vi "code_facade.vi"(0 "Data In":T4, 2 "Display State In":T2, 3 "Container State":T3) -> (6 "Data Out":T4, 7 "Display State Out":T2, 8 "Action":T1)   [LabVIEW 2022 SP3, in "Code.xctl"]
uses:
  Code.xctl
  code_data.ctl
  <vilib>/_xctls/Container State.ctl
  code_state.ctl
  <vilib>/_xctls/Action.ctl
  <vilib>/event_ctls.llb/eventvkey.ctl
  <vilib>/_xctls/XControlSupport.lvlib
panel:
  out "VKey":T5
  in  "Python Code":string
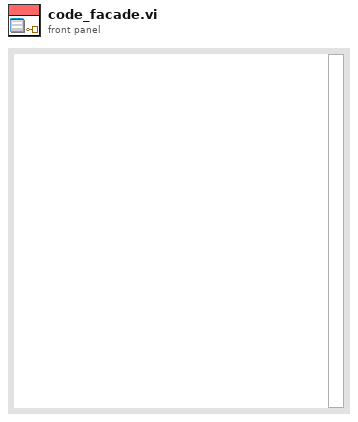
[diagram p1: front panel]
types:
  T1 = typedef "XControlSupport.lvlib/Action.ctl" = cluster{"Data Changed?":bool, "State Changed?":bool, "Action Name":string}
  T2 = typedef "Code.xctl/code_state.ctl" = cluster{"Numeric":dbl}
  T3 = typedef "XControlSupport.lvlib/Container State.ctl" = cluster{"Indicator?":bool, "Run Mode?":bool, " Refnum":refnum<vi>}
  T4 = typedef "Code.xctl/code_data.ctl" = string
  T5 = typedef "eventvkey.ctl" = enum16{"ASCII", "Enter", "Return", "Shift", "Ctrl", "Alt", "Cmd", "Opt", "Caps", "NumLock", "Clear", "Break", "Up", "Down", "Left", "Right", "Insert", "Delete", "Home", "End", "PageUp", "PageDown", "Escape", "Help", "Pause", "ScrollLock", "F1", "F2", "F3", "F4", "F5", "F6", "F7", "F8", "F9", "F10", "F11", "F12", "F13", "F14", "F15", "F16", "F17", "F18", "F19", "F20", "F21", "F22", "F23", "F24", "Play", "VolumeUp", "VolumeDown", "Mute", "Two Byte Char"}
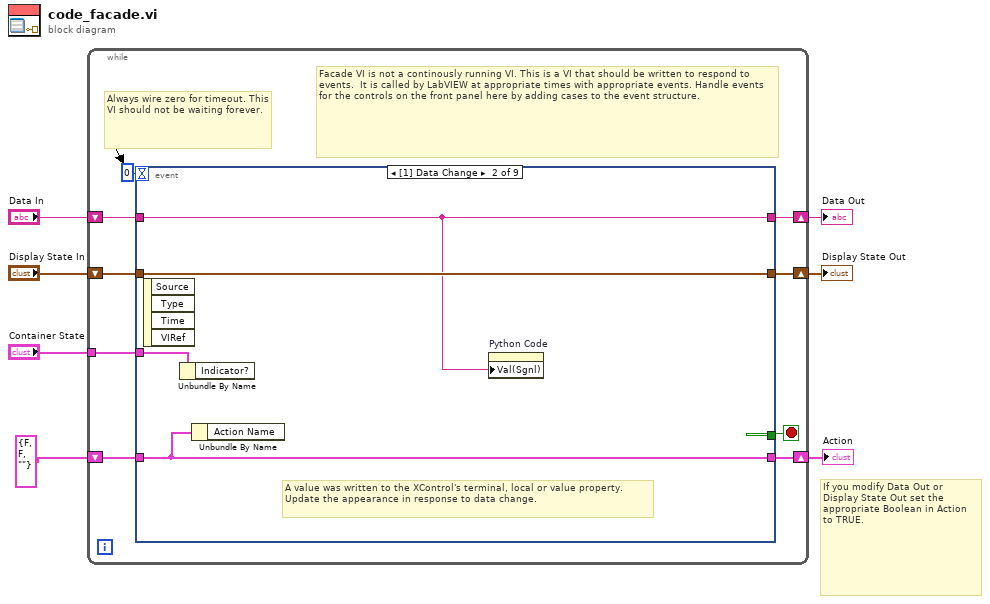
[diagram p0: block diagram]
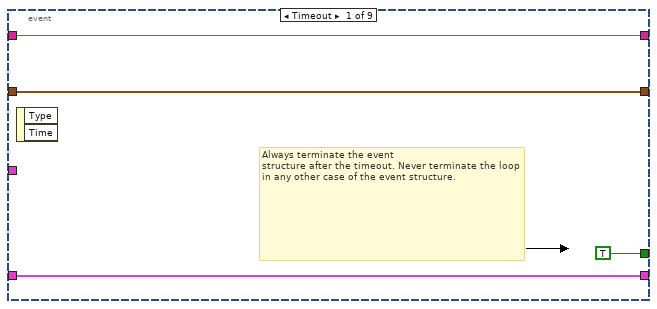
[diagram p2: hidden frame]
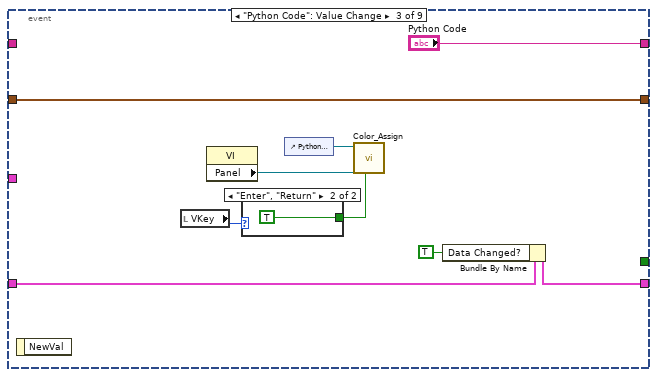
[diagram p3: hidden frame]
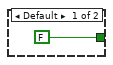
[diagram p4: hidden frame]
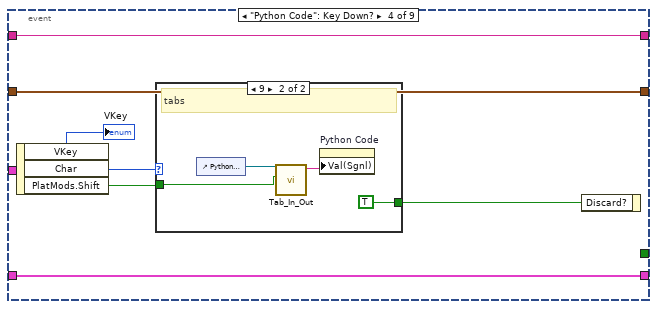
[diagram p5: hidden frame]
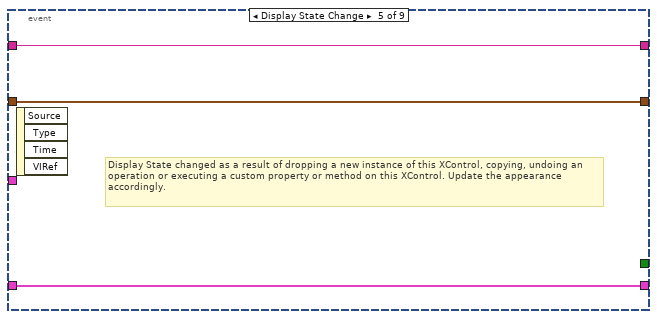
[diagram p7: hidden frame]
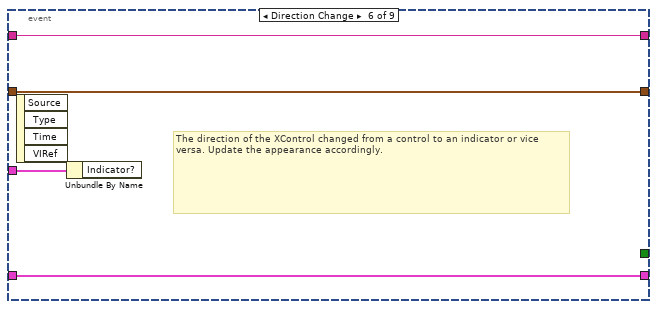
[diagram p8: hidden frame]
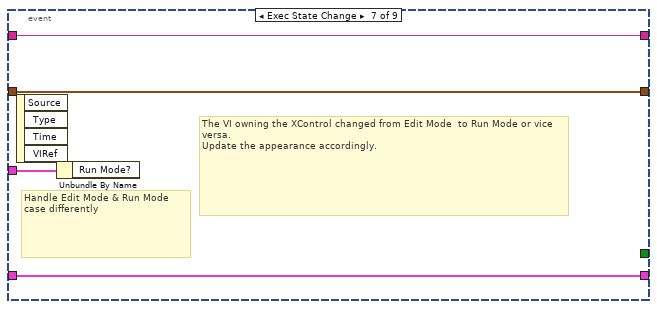
[diagram p9: hidden frame]
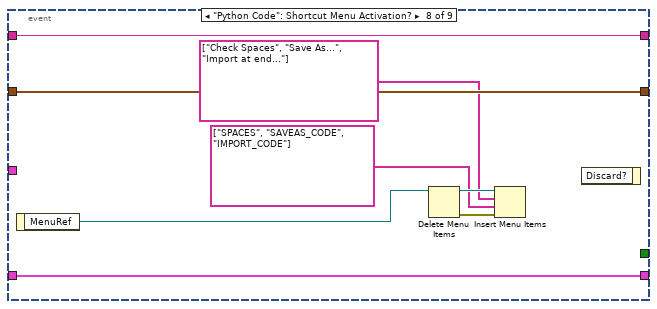
[diagram p10: hidden frame]
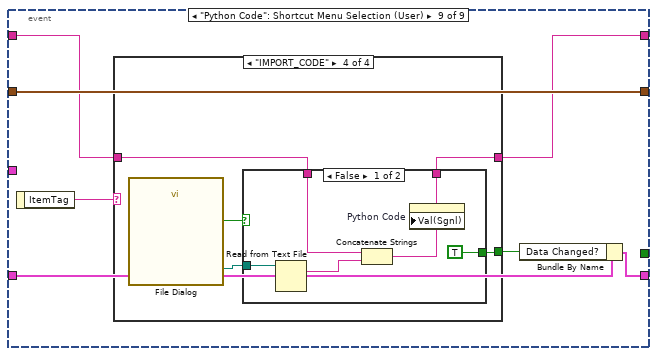
[diagram p11: hidden frame]
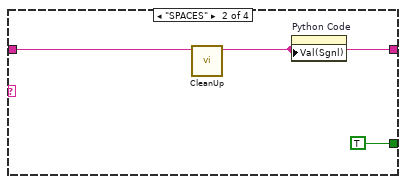
[diagram p13: hidden frame]
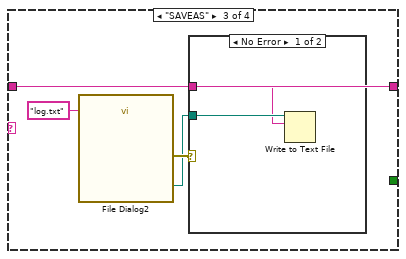
[diagram p14: hidden frame]
diagram:
  # "If you modify Data Out or\nDisplay State Out set the\nappropriate Boolean in Action\nto TRUE."
  n1 = while {
    shift-right: [w15] -> w4
    shift-left: "Display State In" -> [w16]
    tunnel: "Container State" -> [w12]
    shift-right: [w10] -> w7
    shift-left: "Data In" -> [w11]
    shift-right: [w8] -> w2
    shift-left: T1 {"Data Changed?"=FALSE, "State Changed?"=FALSE, "Action Name"=""} ("Action") -> [w9]
    stop <- w14 stop-if-true
    # "Facade VI is not a continously running VI. This is a VI that should be written to respond to events.  It is called by LabVIEW at appropriate times with appropriate events. Handle events for the controls on the front panel here by adding cases to the event structure."
    # "Always wire zero for timeout. This\nVI should not be waiting forever."
    n2 = event shown="[1] Data Change" {
      selector: _ -> [_ _ _ _ _ _ _ _ _]
      dyn-events: _ -> [_ _ _ _ _ _ _ _ _]
      timeout: 0 -> [_ _ _ _ _ _ _ _ _]
      tunnel: w16 -> [w18 w24 w33 w42 w49 w52 w56 w65 w72]
      tunnel: [w18 w24 w33 w42 w49 w52 w56 w65 w72] -> w15
      tunnel: [TRUE _ _ _ _ _ _ _ _] -> w14
      tunnel: w12 -> [_ w23 _ _ _ w53 w57 _ _]
      tunnel: w11 -> [w17 w21 _ w40 w48 w51 w55 w64 w69]
      tunnel: [w17 w21 "Python Code" w40 w48 w51 w55 w64 w70] -> w10
      tunnel: [w19 w22 w30 w41 w47 w50 w54 w63 w67] -> w8
      tunnel: w9 -> [w19 w22 w29 w41 w47 w50 w54 w63 w66]
      event Timeout {
        # "Always terminate the event\nstructure after the timeout. Never terminate the loop in any other case of the event structure."
        n3 = event-data() -> ()  [unwired: 1 in, 2 out]
      }
      event Data Change {
        # "A value was written to the XControl's terminal, local or value property.\nUpdate the appearance in response to data change."
        n4 = event-data() -> ()  [unwired: 1 in, 4 out]
        n5 = Unbundle By Name(w23) -> ()  [unwired: 1 out]
        n6 = Unbundle By Name(w22) -> ()  [unwired: 1 out]
        n7 = property on="Python Code" class="Str"("Val(Sgnl)"=w21) -> ()  [unwired: 2 in, 2 out]
      }
      event "Python Code": Value Change {
        n8 = event-data() -> ()  [unwired: 1 in, 1 out]
        n9 = local read "VKey"() -> (w26:T5)
        n10 = property class="VI"() -> ("Panel"=w31:refnum<vi>)  [unwired: 2 in, 2 out]
        n11 = case shown="\"Enter\", \"Return\"" w26 {
          tunnel: [FALSE TRUE] -> w25
          frame Default {
          }
          frame "Enter", "Return" {
          }
        }
        n12 = control-ref of="Python Code"() -> (w32:refnum<vi>)
        n13 = call "Color_Assign.vi"("Add Spaces?"=w25, "Front Panel"=w31, "Code"=w32) -> ()  [unwired: 8 in, 1 out]
        n14 = Bundle By Name(cluster=w29, "Data Changed?"=TRUE) -> (w30:T1)
      }
      event "Python Code": Key Down? {
        n15 = event-data() -> ("VKey"=→"VKey":T5, "Char"=w39:i16, "PlatMods.Shift"=w38:bool)  [unwired: 1 in]
        n16 = case shown="9" w39 {
          tunnel: w38 -> [_ w44]
          tunnel: [_ TRUE] -> w36
          frame 0, Default {
          }
          frame 9 {
            # "tabs"
            n17 = control-ref of="Python Code"() -> (w45:refnum<vi>)
            n18 = call "Tab_In_Out.vi"("Shift?"=w44, "String in"=w45) -> ("result string"=w46:string)  [unwired: 9 in]
            n19 = property on="Python Code" class="Str"("Val(Sgnl)"=w46) -> ()  [unwired: 2 in, 2 out]
          }
        }
        n20 = event-data("Discard?"=w36) -> ()  [unwired: 1 in, 1 out]
      }
      event Display State Change {
        # "Display State changed as a result of dropping a new instance of this XControl, copying, undoing an operation or executing a custom property or method on this XControl. Update the appearance accordingly."
        n21 = event-data() -> ()  [unwired: 1 in, 4 out]
      }
      event Direction Change {
        # "The direction of the XControl changed from a control to an indicator or vice versa. Update the appearance accordingly."
        n22 = event-data() -> ()  [unwired: 1 in, 4 out]
        n23 = Unbundle By Name(w53) -> ()  [unwired: 1 out]
      }
      event Exec State Change {
        # "The VI owning the XControl changed from Edit Mode  to Run Mode or vice versa.\nUpdate the appearance accordingly."
        # "Handle Edit Mode & Run Mode\ncase differently"
        n24 = event-data() -> ()  [unwired: 1 in, 4 out]
        n25 = Unbundle By Name(w57) -> ()  [unwired: 1 out]
      }
      event "Python Code": Shortcut Menu Activation? {
        n26 = event-data() -> ("MenuRef"=w58:refnum<k9>)  [unwired: 1 in]
        n27 = Delete Menu Items(9:w58) -> (0:w62:errorcluster, 3:w61:refnum<k9>)  [unwired: 3 in]
        n28 = Insert Menu Items(6:w62, 7:string[] ["SPACES", "SAVEAS_CODE", "IMPORT_CODE"], 8:string[] ["Check Spaces", "Save As...", "Import at end..."] ("L10n_Parent Menus"), 9:w61) -> ()  [unwired: 2 in, 3 out]
        n29 = event-data() -> ()  [unwired: 2 in, 1 out]
      }
      event "Python Code": Shortcut Menu Selection (User) {
        n30 = event-data() -> ("ItemTag"=w71:string)  [unwired: 1 in]
        n31 = case shown="\"IMPORT_CODE\"" w71 {
          tunnel: w69 -> [w73 w76 w77 w85]
          tunnel: [w73 w74 w77 w84] -> w70
          tunnel: [_ TRUE ("Data Changed?") _ w83] -> w68
          frame Default {
          }
          frame "SPACES" {
            n32 = call "CleanUp.vi"("Python Code"=w76) -> ("spreadsheet string"=w74:string)  [unwired: 10 in]
            n33 = property on="Python Code" class="Str"("Val(Sgnl)"=w74) -> ()  [unwired: 2 in, 2 out]
          }
          frame "SAVEAS" {
            n34 = call "File Dialog2"("default name"="log.txt") -> ("selected path"=w79:path, "error out"=w80:errorcluster)  [unwired: 11 in, 2 out]
            n35 = case shown="No Error" w80 {
              tunnel: w79 -> [w82 _]
              tunnel: w77 -> [w81 _]
              frame No Error {
                n36 = Write to Text File(file (use dialog)=w82, text=w81) -> ()  [unwired: 2 in, 3 out]
              }
              frame Error {
              }
            }
          }
          frame "IMPORT_CODE" {
            n37 = call "File Dialog"() -> ("selected path"=w86:path, "cancelled"=w87:bool)  [unwired: 12 in, 2 out]
            n38 = case shown="False" w87 {
              tunnel: w86 -> [w92 _]
              tunnel: w85 -> [w90 w93]
              tunnel: [w88 w93] -> w84
              tunnel: [TRUE _] -> w83
              frame False {
                n39 = Read from Text File(file (use dialog)=w92) -> (text=w91:string)  [unwired: 3 in, 3 out]
                n40 = Concatenate Strings(w90, w91) -> (w88:string)
                n41 = property on="Python Code" class="Str"("Val(Sgnl)"=w88) -> ()  [unwired: 2 in, 2 out]
              }
              frame True {
              }
            }
          }
        }
        n42 = Bundle By Name(cluster=w66, "Data Changed?"=w68) -> (w67:T1)
      }
    }
  }
  "Display State Out" <- w4
  "Data Out" <- w7
  "Action" <- w2
